vi "Obtain CTRL Data Notifier.vi"(8 "error in (no error)":errorcluster) -> (0 "error out":errorcluster, 3 "CTRL Data Notifier out":refnum<notifier>)   [LabVIEW 2014, in "WINFAS 2 Data Queue.lvlib"]
uses:
  WINFAS 2 Data Queue.lvlib
  Control Data Cluster.ctl
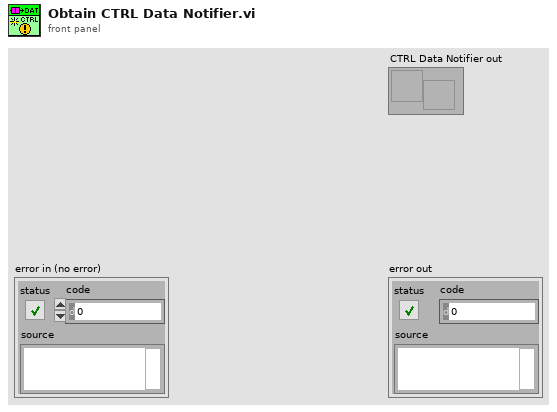
[diagram p1: front panel]
types:
  T1 = typedef "WINFAS 2 Data Queue.lvlib/Control Data Cluster.ctl" = cluster{"Encoder":sgl, "DI":bool[], "DO":bool[]}
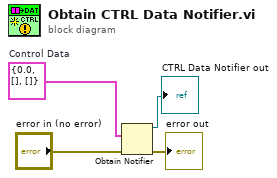
[diagram p0: block diagram]
diagram:
  w2 = T1 {"Encoder"=0.0, "DI"=[], "DO"=[]}  # Control Data
  n1 = Obtain Notifier(notification data type=w2, error in (no error)="error in (no error)") -> (notifier out=→"CTRL Data Notifier out":refnum<notifier>, error out=→"error out":errorcluster)  [unwired: 2 in, 1 out]
